vi "Handle Invalid NaN.vi"(11 "String":string) -> (3 "result string":string)   [LabVIEW 2019, in "LV-Data.PGSQL.lvclass"]
uses:
  LV-Data.PGSQL.lvclass
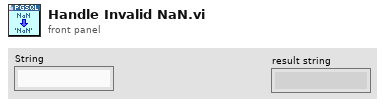
[diagram p1: front panel]
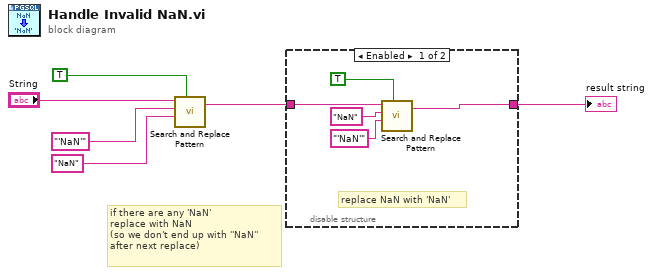
[diagram p0: block diagram]
diagram:
  # "if there are any 'NaN'\nreplace with NaN\n(so we don't end up with ''NaN''\nafter next replace)"
  n1 = call <vilib>:"Search and Replace Pattern.vi"("string"="String", "regular expression (\"\")"="'NaN'" ("regular expression (\"\")"), "replace string (\"\")"="NaN" ("replace string (\"\")"), "replace all? (F)"=TRUE) -> ("result string"=w5:string)  [unwired: 1 in, 1 out]
  n2 = disable-structure shown="Enabled" {
    disable-tunnel: [w11 w12] -> w6
    disable-tunnel: w5 -> [w10 w12]
    frame Enabled {
      # "replace NaN with 'NaN'"
      n3 = call <vilib>:"Search and Replace Pattern.vi"("string"=w10, "regular expression (\"\")"="NaN" ("regular expression (\"\")"), "replace string (\"\")"="'NaN'" ("replace string (\"\")"), "replace all? (F)"=TRUE) -> ("result string"=w11:string)  [unwired: 1 in, 1 out]
    }
    frame Disabled {
    }
  }
  "result string" <- w6
